vi "TimeTag_LSW_edits_June18.vi"() -> ()   [LabVIEW 2015]
doc: "This sample project is built upon the standard state machine template and shows how you could create an application that acquires, analyzes, and presents data. It includes functionality for presenting configuration dialogs, preserving settings between executions, loading and saving data, as well as exporting graph images and text files.\n\nIt is most appropriate for data that is acquired instantly as it does not allow for screen updates mid acquisition nor does it allow for continuous streaming to disk."
uses:
  <vilib>/ptbypt/NI_PtbyPt.lvlib
panel:
  out "Total Ch2 CPS":dbl
  out "Total Ch4 CPS":dbl
  in  "Averaging":dbl
  in  "Runs":dbl=100.0
  in  "Pulse TTL 2":bool
  in  "Pulse TTL 1":bool
  in  "Toggle\nTTL 2":bool
  in  "Toggle\nTTL 1":bool
  out "Total Starts":dbl
  in  "Record data":bool
  out "Initial time":dbl
  out "Elapsed time (s)":dbl
  out "FPGA_Run Status":dbl
  out "USB_Open Status":dbl
  out "Channel 4 Total\nCounts":dbl
  out "Channel 3 Total\nCounts":dbl
  out "Channel 2 Total\nCounts":dbl
  out "Channel 1 Total\nCounts":dbl
  in  "File Name":string="C:\\FPGA\\test.txt"
  out "?":dbl
  out "?":dbl
  out "?":dbl
  out "?":dbl
  out "stats":i64[](array[numeric])
  in  "Stop":bool
  out "Channel 4 CPS":dbl(knob) scale=0.0..700.0
  out "Channel 3 CPS":dbl(knob) scale=0.0..600.0
  out "Channel 2 CPS":dbl(knob) scale=0.0..700.0
  out "Channel 1 CPS":dbl(knob) scale=0.0..600.0
  # "Starts"
  # "Channel 1"
  # "Channel 2"
  # "Channel 3"
  # "Channel 4"
  # "Coincidence Channels 1 & 2"
  # "Coincidence Channels 1 & 3"
  # "Coincidence Channels 1 & 4"
  # "Coincidence Channels 2 & 3"
  # "Coincidence Channels 2 & 4"
  # "Coincidence Channels 3 & 4"
  # "Coincidence Channels 1 & 2 & 3"
  # "Coincidence Channels 1 & 2 & 4"
  # "Coincidence Channels 1 & 3 & 4"
  # "Coincidence Channels 2 & 3 & 4"
  # "Coincidence Channels 1 & 2 & 3 & 4"
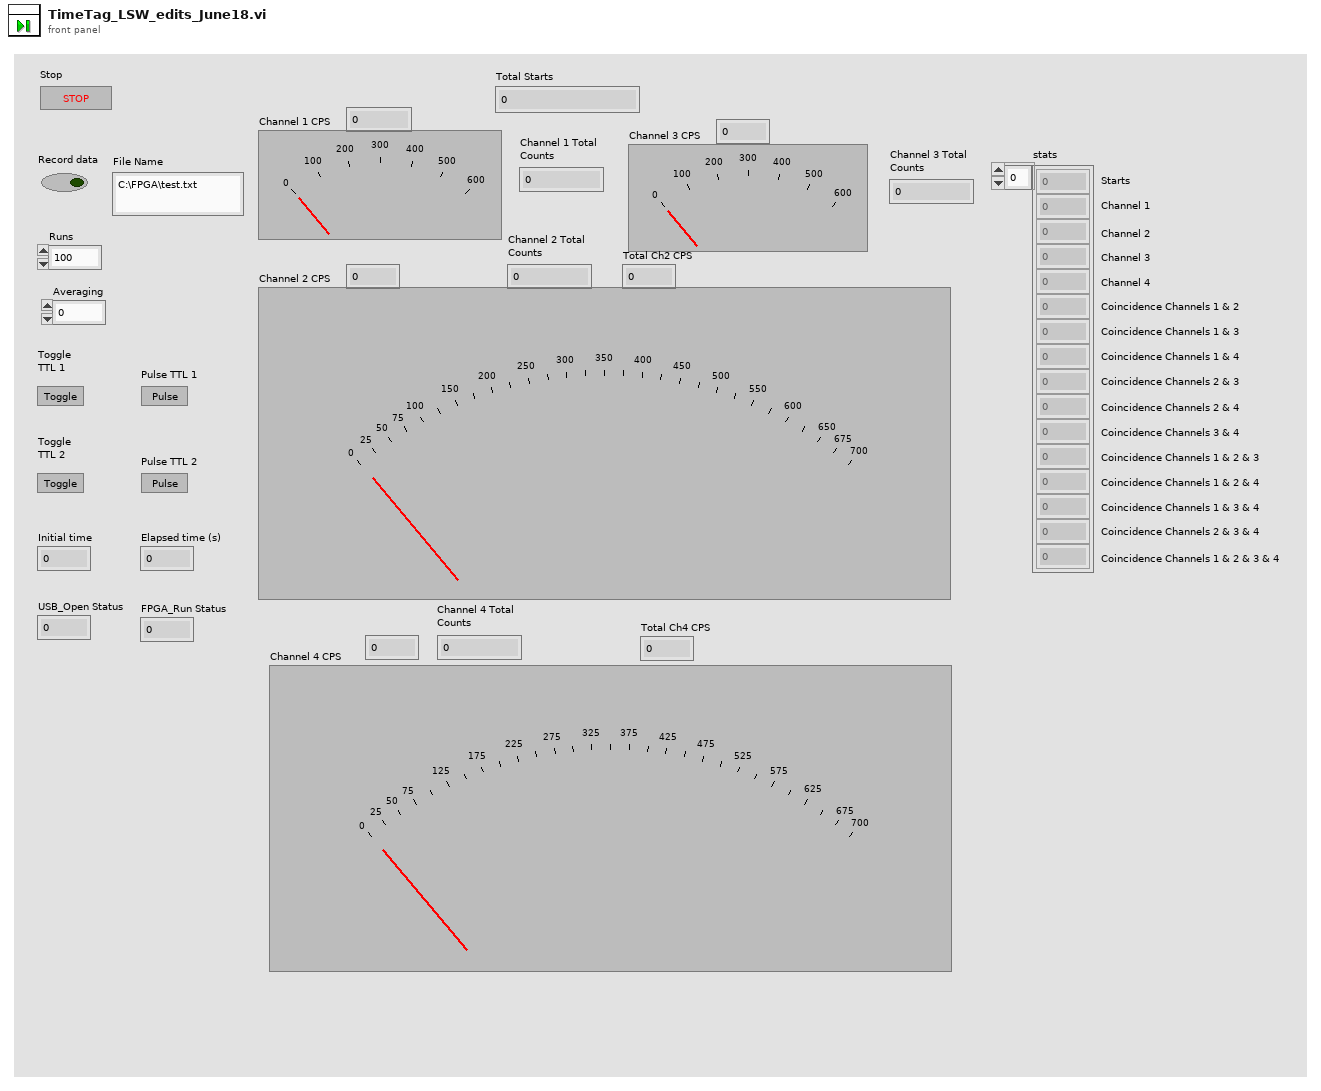
[diagram p1: front panel]
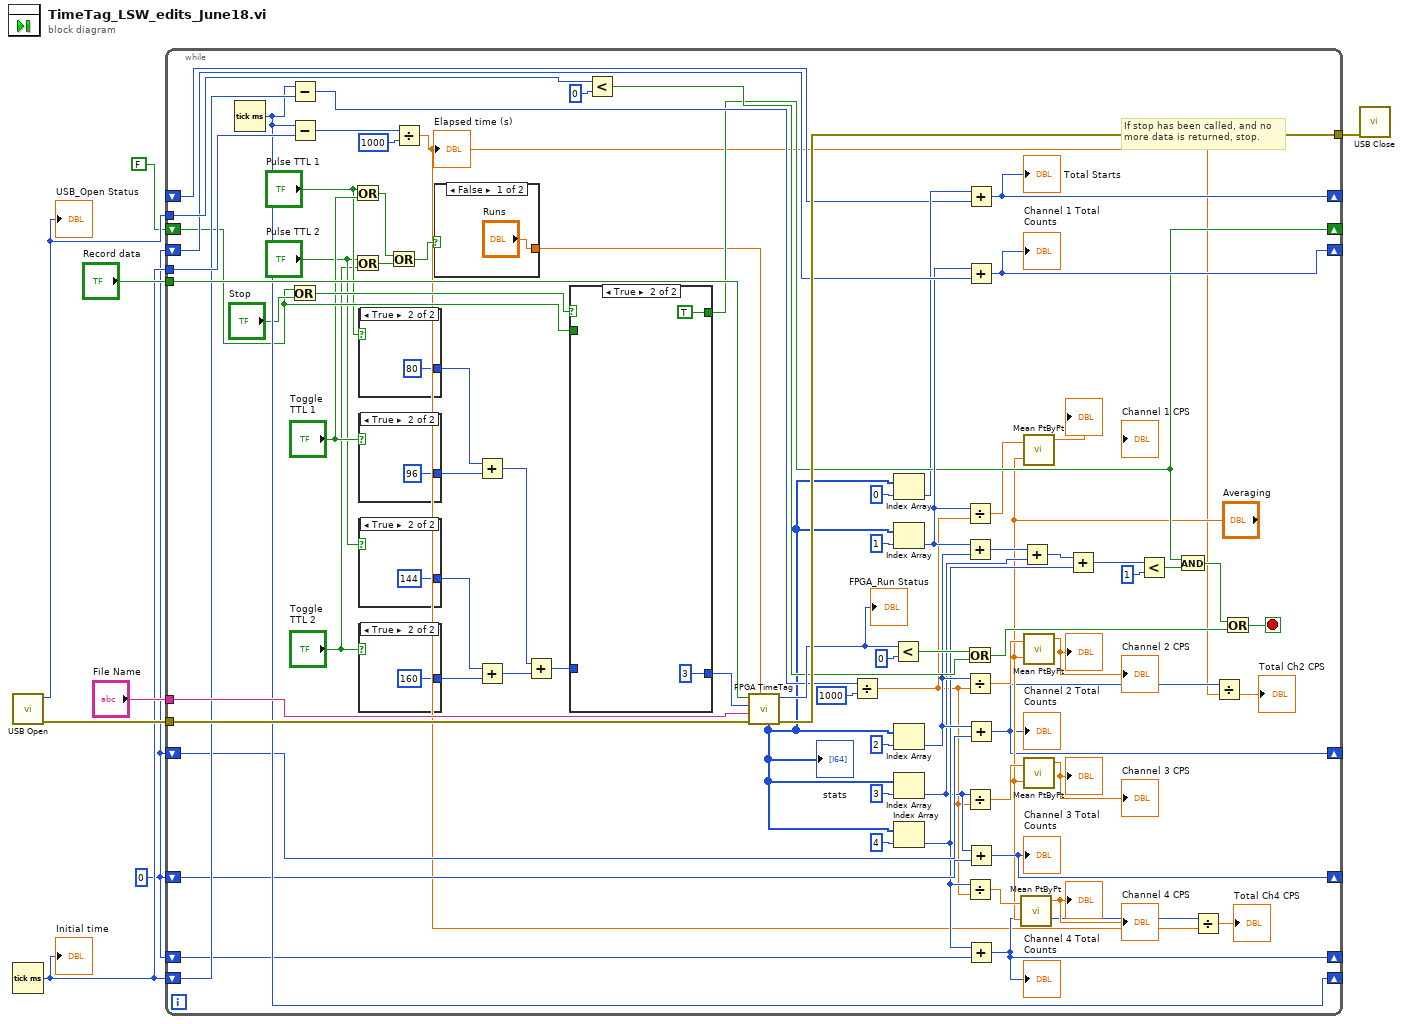
[diagram p0: block diagram]
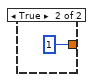
[diagram p2: hidden frame]
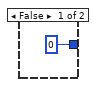
[diagram p3: hidden frame]
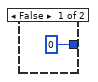
[diagram p4: hidden frame]
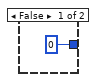
[diagram p5: hidden frame]
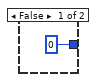
[diagram p6: hidden frame]
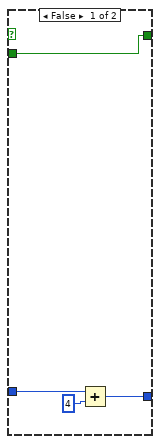
[diagram p7: hidden frame]
diagram:
  w2 = 0
  n1 = call "USB Open.vi"() -> ("error out"=w6:errorcluster, "function return"=w3:i32)  [unwired: 10 in]
  "USB_Open Status" <- w3
  n2 = Tick Count (ms)() -> (millisecond timer value=w4:u32)
  "Initial time" <- w4
  n3 = while {
    tunnel: w4 -> [w87]
    shift-right: [w65] -> _
    shift-left: w2 -> [w61]
    shift-right: [w12] -> _
    shift-left: w2 -> [w60]
    shift-right: [w64] -> _
    shift-left: w2 -> [w59]
    shift-right: [w13] -> _
    shift-left: w2 -> [w58]
    tunnel: w6 -> [w77]
    tunnel: [w78] -> w5
    tunnel: "Record data" -> [w75]
    tunnel: "File Name" -> [w76]
    shift-right: [w62] -> _
    shift-left: w4 -> [w73]
    tunnel: w3 -> [w69]
    shift-right: [w47] -> _
    shift-left: FALSE -> [w44]
    shift-right: [w38] -> _
    shift-left: _ -> [w40]
    stop <- w79 stop-if-true
    # "If stop has been called, and no\nmore data is returned, stop."
    n4 = Tick Count (ms)() -> (millisecond timer value=w62:u32)
    n5 = Subtract(x=w62, y=w73) -> (x-y=w72:u32)
    n6 = Subtract(x=w62, y=w87) -> (x-y=w86:u32)
    n7 = Or(x=w44, y="Stop") -> (x .or. y?=w46:bool)
    n8 = Or(x="Pulse TTL 1", y="Toggle\nTTL 1") -> (x .or. y?=w29:bool)
    n9 = Or(x="Pulse TTL 2", y="Toggle\nTTL 2") -> (x .or. y?=w30:bool)
    n10 = case shown="True" "Pulse TTL 1" {
      tunnel: [0 80] -> w37
      frame False {
      }
      frame True {
      }
    }
    n11 = case shown="True" "Toggle\nTTL 1" {
      tunnel: [0 96] -> w36
      frame False {
      }
      frame True {
      }
    }
    n12 = case shown="True" "Pulse TTL 2" {
      tunnel: [0 144] -> w33
      frame False {
      }
      frame True {
      }
    }
    n13 = case shown="True" "Toggle\nTTL 2" {
      tunnel: [0 160] -> w34
      frame False {
      }
      frame True {
      }
    }
    n14 = Or(x=w29, y=w30) -> (x .or. y?=w31:bool)
    n15 = Divide(x=w86, y=1000) -> (x/y=w11:dbl)
    "Elapsed time (s)" <- w11
    n16 = case shown="False" w31 {
      tunnel: ["Runs" 1] -> w27
      frame False {
      }
      frame True {
      }
    }
    n17 = Add(x=w37, y=w36) -> (x+y=w35:i32)
    n18 = Add(x=w33, y=w34) -> (x+y=w32:i32)
    n19 = Add(x=w35, y=w32) -> (x+y=w28:i32)
    n20 = case shown="True" w46 {
      tunnel: [w99 3] -> w63
      tunnel: [w101 TRUE] -> w47
      tunnel: w44 -> [w101 _]
      tunnel: w28 -> [w98 _]
      frame False {
        n21 = Add(x=w98, y=4) -> (x+y=w99:i32)
      }
      frame True {
      }
    }
    n22 = Less?(x=w69, y=0) -> (x < y?=w67:bool)
    n23 = call "FPGA TimeTag.vi"("runs"=w27, "error in (no error)"=w77, "fileName"=w76, "fpgaCommand"=w63, "saveData"=w75) -> ("error out"=w78:errorcluster, "function return"=w74:i32, "stats"=w41:i64[])  [unwired: 4 in]
    "stats" <- w41
    "FPGA_Run Status" <- w74
    n24 = Divide(x=w72, y=1000) -> (x/y=w39:dbl)
    n25 = Less?(x=w74, y=0) -> (x < y?=w68:bool)
    n26 = Index Array(array=w41, index=0) -> (element=w42:i64)
    n27 = Index Array(array=w41, index=1) -> (element=w50:i64)
    n28 = Index Array(array=w41, index=2) -> (element=w57:i64)
    n29 = Index Array(array=w41, index=3) -> (element=w53:i64)
    n30 = Index Array(array=w41, index=4) -> (element=w54:i64)
    n31 = Divide(x=w50, y=w39) -> (x/y=w22:dbl)
    n32 = Add(x=w50, y=w57) -> (x+y=w52:i64)
    n33 = Or(x=w68, y=w67) -> (x .or. y?=w66:bool)
    n34 = Divide(x=w57, y=w39) -> (x/y=w21:dbl)
    n35 = Divide(x=w53, y=w39) -> (x/y=w20:dbl)
    n36 = Divide(x=w54, y=w39) -> (x/y=w18:dbl)
    n37 = Add(x=w42, y=w40) -> (x+y=w38:i64)
    "Total Starts" <- w38
    n38 = Add(x=w50, y=w61) -> (x+y=w65:i64)
    "Channel 1 Total\nCounts" <- w65
    n39 = Add(x=w57, y=w60) -> (x+y=w12:i64)
    "Channel 2 Total\nCounts" <- w12
    n40 = Add(x=w53, y=w59) -> (x+y=w64:i64)
    "Channel 3 Total\nCounts" <- w64
    n41 = Add(x=w54, y=w58) -> (x+y=w13:i64)
    "Channel 4 Total\nCounts" <- w13
    n42 = call <vilib>:"Mean PtByPt.vi"("x"=w18, "sample length"="Averaging") -> ("mean"=→"Channel 4 CPS" →"?":dbl)  [unwired: 2 in, 1 out]
    n43 = Add(x=w52, y=w53) -> (x+y=w56:i64)
    n44 = call <vilib>:"Mean PtByPt.vi"("x"=w22, "sample length"="Averaging") -> ("mean"=→"?":dbl)  [unwired: 2 in, 1 out]
    n45 = call <vilib>:"Mean PtByPt.vi"("x"=w21, "sample length"="Averaging") -> ("mean"=→"Channel 2 CPS" →"?":dbl)  [unwired: 2 in, 1 out]
    n46 = call <vilib>:"Mean PtByPt.vi"("x"=w20, "sample length"="Averaging") -> ("mean"=→"Channel 3 CPS" →"?":dbl)  [unwired: 2 in, 1 out]
    n47 = Add(x=w56, y=w54) -> (x+y=w55:i64)
    n48 = Less?(x=w55, y=1) -> (x < y?=w49:bool)
    n49 = And(x=w47, y=w49) -> (x .and. y?=w48:bool)
    n50 = Divide(x=w13, y=w11) -> (x/y=→"Total Ch4 CPS":dbl)
    n51 = Divide(x=w12, y=w11) -> (x/y=→"Total Ch2 CPS":dbl)
    n52 = Or(x=w48, y=w66) -> (x .or. y?=w79:bool)
  }
  n53 = call "USB Close.vi"("error in (no error)"=w5) -> ()  [unwired: 9 in, 2 out]
